vi "Initialize Target Project.vi"(8 "error in (no error)":errorcluster, 11 "ComboBox in":refnum<vi>) -> (0 "error out":errorcluster, 2 "Projects":T1)   [LabVIEW 2019, in "Configuration Tool.lvlib"]
uses:
  Configuration Tool.lvlib
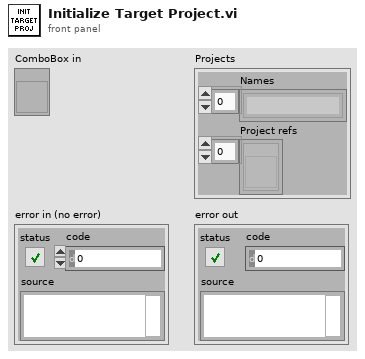
[diagram p1: front panel]
types:
  T1 = cluster{"Names":string[], "Project refs":refnum<vi>[]}
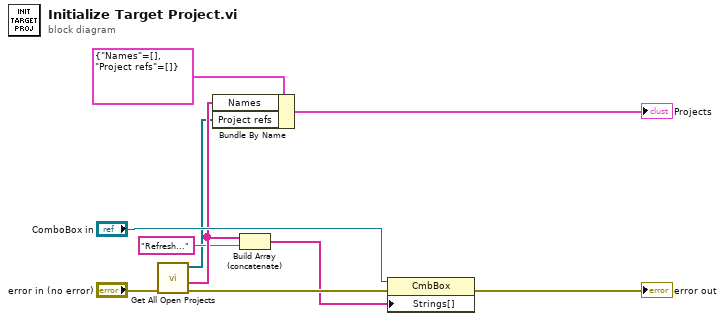
[diagram p0: block diagram]
diagram:
  n1 = call "Get All Open Projects.vi"("error in (no error)"="error in (no error)") -> ("error out"=w10:errorcluster, "Names"=w4:string[], "Project refs out"=w1:refnum<vi>[])  [unwired: 8 in]
  n2 = Bundle By Name(cluster=T1 {"Names"=[], "Project refs"=[]}, "Names"=w4, "Project refs"=w1) -> (→"Projects":T1)
  n3 = Build Array (concatenate)(w4, "Refresh..." ("Name")) -> (w2:string[])
  n4 = property on="Property Node" class="CmbBox"(reference="ComboBox in", error in=w10, "Strings[]"=w2) -> (error out=→"error out":errorcluster)  [unwired: 1 out]
